vi "Tetra_TX-PROD_Setup.vi"() -> (0 "error out":errorcluster, 2 "Status":string="Skipping Setup of Power Supply\rDone !!!\rDONE!!\n\nSetting up PNA...\rRecalling PNA Setup:  Z:\\State Files\\TEST2.csa\rDONE!!!\rSkipping Spectrum Analyzer!!!\rSkipping Setting Up Temperature...\rSetup Complete !!!")   [LabVIEW 2018]
uses:
  <vilib>/Utility/error.llb/DialogType.ctl
  Tetra_Globals.vi
  Initialize References/Sequence Globals.vi
  Infrastructure/Test Parameter Globals_1.0.0.vi
  Initialize References/Station References Global.vi
  Infrastructure/Test Result File Name Global.vi
  <vilib>/Utility/file.llb/Read Delimited Spreadsheet (string).vi
  <vilib>/Utility/file.llb/Write Delimited Spreadsheet (string).vi
  Instruments/PNA/lib functions/Agilent ENA Series.lvlib
  Instruments/Agilent N5232A PNA-L/Labview Driver/Keysight PNA Series/Keysight PNA Series.lvlib
panel:
  out "IsPSA?(t)":bool
  out "Meas_S11?(t)":bool
  out "OUT_CAL_PATH(str)":string
  in  "ess_error":errorcluster
  in  "Tab Control":T1(tab)
  in  "Setup Chip (T)":bool=TRUE
  in  "Setup Power Supply (T)":bool=TRUE
  in  "Setup PNA (T)":bool=TRUE
  in  "Kill Teraterm":bool=TRUE
  in  "Setup Gantry(t)":bool=TRUE
  in  "Setup EXA(t)":bool=TRUE
  out "Success":bool
  out "MODE":bool
  out "COM PORT":string="COM4"
  out "RBW":string="3000"
  out "Avgs":u32=4
  out "SPAN":dbl=0.1
  out "REF_LVL":dbl=10.0
  out "PS1-1(V)":dbl=18.75
  out "PS1-1(A)":dbl=1.0
  out "PS1-2(V)":dbl=5.0
  out "PS1-2(A)":dbl=1.0
  out "Use PS1-2":bool=TRUE
  out "Use PS1-1":bool=TRUE
  out "EXA State File":string="Z:\\State Files\\State_0000.state"
  out "cmd;":string
  out "ATT_LVL":dbl=10.0
  out "TEMP":dbl=25.0
  out "TEMP?(t)":bool
  out "RF_FREQ":dbl=20.0
  out "f_ref":dbl=10.0
  out "REF_POWER":dbl=7.5
  out "Soak Time (s)":dbl=10.0 caption="Delay Time (s)"
  out "Ant":i16
  out "Gantry-Z":dbl
  out "GET_DET":bool
  out "OUT_CAL_PATH":path=path "C:/RageATE/Automated Tests/Tetra WAM/DVT/Cal Files/OUTPUT_CAL_080321-1118.csv"
  out "HORN_CAL_PATH":path
  out "RF_CAL_PATH":path
  out "git log":string="#RageATE gitlog: commit 9dda47de5732cf8fa6a9554b7d9ab91f125b5971\n#RageATE gitlog: Author: rick-rage <rick@ragesystems.com>\n#RageATE gitlog: Date:   Mon Aug 2 15:21:18 2021 -0400\n#RageATE gitlog: This Computer Name : CRANES\r\n\r\n"
  out "PNA State File":string="Z:\\State Files\\TEST2.csa"
  out "Text":refnum<vi>
  out "s11_path":path
  out "Pmic_FwRev":string
  out "i_mon":string
  out "rev":string="rdiv\r\n0)  sw3p6:   195 mA  3616 mV\r\n1)  sw5p5:    89 mA  5472 mV\r\n2) sw2p8a:   315 mA  2784 mV\r\n3) sw2p8b:   349 mA  2768 mV\r\n4)  sw2p4:  1458 mA  2288 mV\r\n5)  sw1p4:  1047 mA  1304 mV\r\n>"
  out "snic":string="#Family: 0x2D\n#Serial: 0x000036092740\r\n"
  in  "error in (no error)":errorcluster
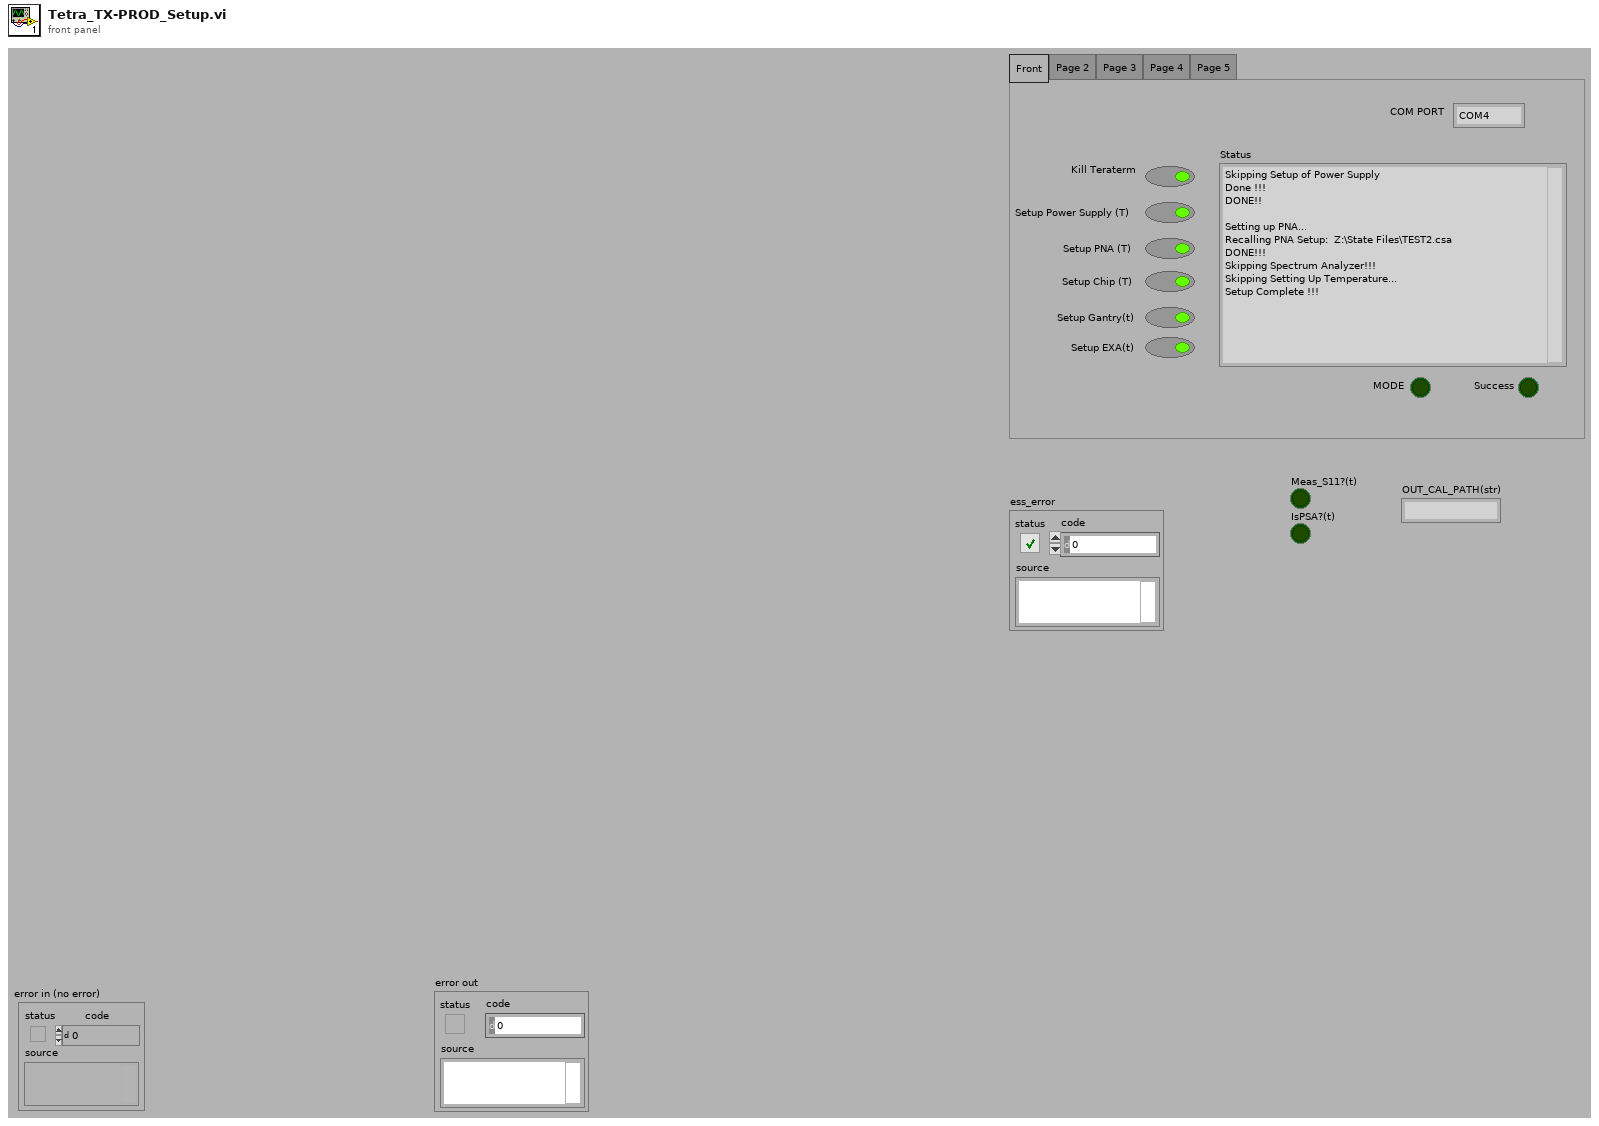
[diagram p1: front panel]
types:
  T1 = enum32{"Front", "Page 2", "Page 3", "Page 4", "Page 5"}
  T2 = typedef "DialogType.ctl" = u16
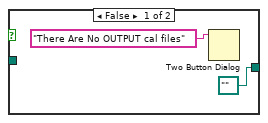
[diagram p2: hidden frame]
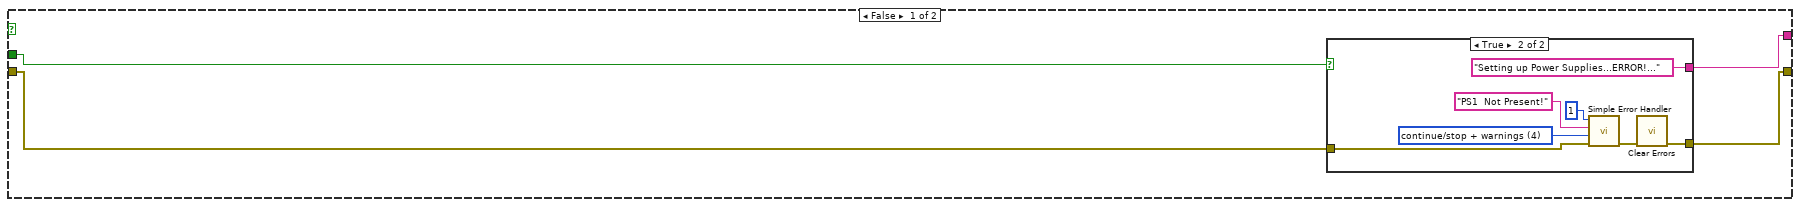
[diagram p6: hidden frame]
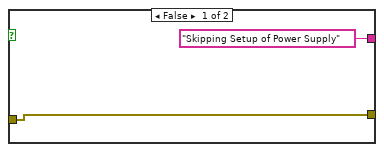
[diagram p7: hidden frame]
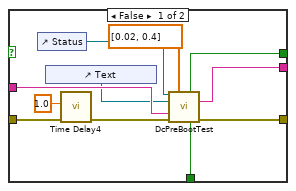
[diagram p8: hidden frame]
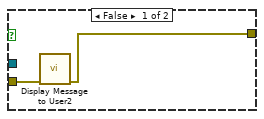
[diagram p10: hidden frame]
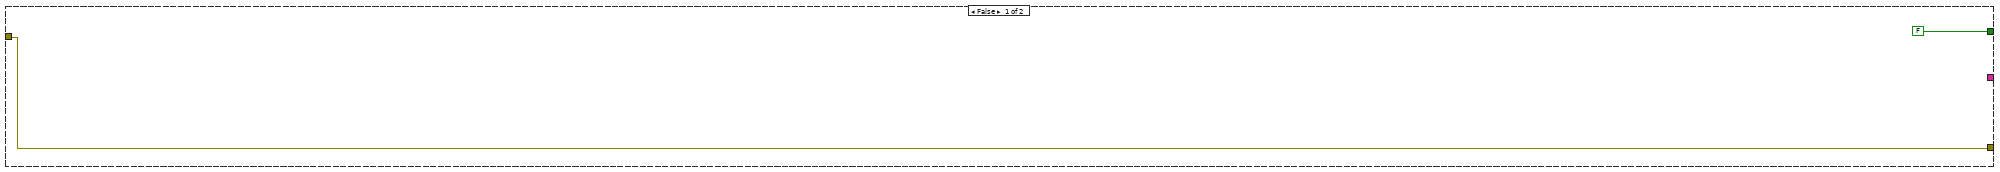
[diagram p11: hidden frame]
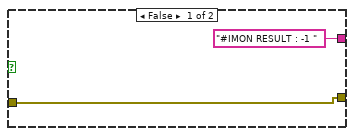
[diagram p12: hidden frame]
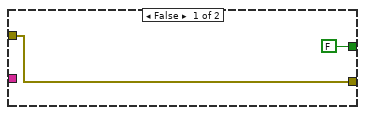
[diagram p13: hidden frame]
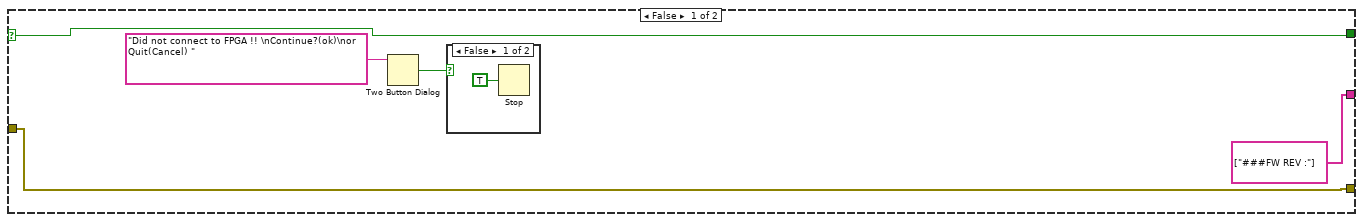
[diagram p14: hidden frame]
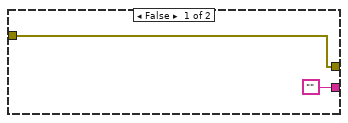
[diagram p16: hidden frame]
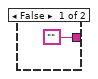
[diagram p18: hidden frame]
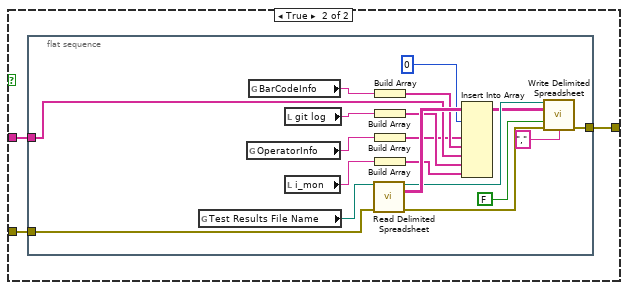
[diagram p19: hidden frame]
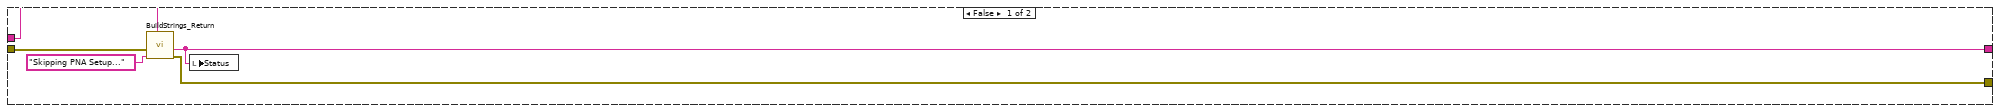
[diagram p20: hidden frame]
diagram:
  n1 = flat-sequence {
    tunnel: [w11] -> w1
    tunnel: [w51] -> w5
    tunnel: [w50] -> w4
    tunnel: w1 -> [w46]
    tunnel: w5 -> [w114]
    tunnel: w4 -> [w113]
    tunnel: [w265] -> w7
    tunnel: [w263] -> w6
    tunnel: w7 -> [w442]
    tunnel: w6 -> [w440]
    tunnel: [w436] -> w2
    tunnel: [w568] -> w3
    tunnel: w2 -> [w571]
    tunnel: w3 -> [w660]
    tunnel: [w655] -> w9
    tunnel: [w659] -> w8
    tunnel: w9 -> [w698]
    tunnel: w8 -> [w701]
    frame #0 {
      # "Kill TeraTerm"
      n2 = flat-sequence {
        tunnel: [w31] -> w11
        frame #0 {
          w29 = 1 items=["INPUT", "OUTPUT"] ("line index")
          (unwired) path "C:/RageATE/Automated Tests/Tetra WAM/PRODUCTION/Test Benches" ("base path")
          n3 = global read "Sequence Globals.vi" "DevSupportPath"() -> (w22:path)
          n4 = Strip Path(path=w22) -> (stripped path=w21:path)  [unwired: 1 out]
          n5 = Build Path(base path=w21, name or relative path=path "Automated Tests/Tetra WAM/PRODUCTION/Test Benches" ("base path")) -> (appended path=w19:path)
          n6 = global read "Sequence Globals.vi" "AppSupportPath"() -> (w25:path)
          n7 = global read "Tetra_Globals.vi" "TestBench_ID"() -> (w23:string)
          n8 = global read "Sequence Globals.vi" "IsRuntime?"() -> (w18:bool)
          n9 = Build Path(base path=w19, name or relative path=w23) -> (appended path=w33:path)
          n10 = Concatenate Strings(w23, " Calibration Files" ("name or relative path")) -> (w24:string)
          n11 = Build Path(base path=w33, name or relative path=w24) -> (appended path=w27:path)
          n12 = Select(t=w25, s=w18, f=w27) -> (s? t:f=w26:path)
          n13 = call "FindMostRecentCalFile.vi"("DIR_IN"=w26, "Test Bench (for filename match)"=w23, "line index"=w29, "IsRuntime?"=w18) -> ("Success?(t)"=w30:bool, "cal_path_out"=w28:path)  [unwired: 9 in, 1 out]
          n14 = case shown="True" w30 {
            tunnel: w28 -> [_ w36]
            tunnel: [path "" ("appended path") w36] -> w31
            frame False {
              n15 = Two Button Dialog(message="There Are No OUTPUT cal files") -> ()  [unwired: 2 in, 1 out]
            }
            frame True {
            }
          }
        }
      }
      n16 = global read "Sequence Globals.vi" "RageATE_Gitlog"() -> (→"git log":string)
      n17 = case shown="True" "Kill Teraterm" {
        tunnel: "error in (no error)" -> [w37 w39]
        tunnel: [w37 w38] -> w13
        tunnel: "taskkill /f /im ttermpro.exe" ("command line") -> [_ w41]
        frame False {
        }
        frame True {
          n18 = call <vilib>:"Clear Errors.vi"("error in (no error)"=w39) -> ("error out"=w40:errorcluster)  [unwired: 5 in, 1 out]
          n19 = call <vilib>:"System Exec.vi"("error in (no error)"=w40, "command line"=w41) -> ("error out"=w42:errorcluster)  [unwired: 6 in, 3 out]
          n20 = call "Time Delay2"("error in (no error)"=w42) -> ("error out"=w38:errorcluster)  [unwired: 10 in]
        }
      }
      n21 = property on="Status" class="Str"(error in=w13) -> (error out=w12:errorcluster, "Text"=→"Text":refnum<vi>)  [unwired: 1 in, 1 out]
      n22 = local write "error in (no error)"(w12) -> ()
    }
    frame #1 {
      n23 = local write "Success"(FALSE ("Success")) -> ()
      n24 = Path To String(path=w46) -> (string=w45:string)
      n25 = local write "Setup EXA(t)"("Setup EXA(t)") -> ()
      n26 = local write "Setup Gantry(t)"("Setup Gantry(t)") -> ()
      n27 = local write "Setup Chip (T)"("Setup Chip (T)") -> ()
      n28 = local write "Setup PNA (T)"("Setup PNA (T)") -> ()
      n29 = Concatenate Strings("#Out_Cal_Path: " ("string"), w45) -> (→"OUT_CAL_PATH(str)":string)
      n30 = local write "Setup Power Supply (T)"("Setup Power Supply (T)") -> ()
      n31 = global read "Test Parameter Globals_1.0.0.vi" "Input Constants Out"() -> (w51:string[])
      n32 = global read "Test Parameter Globals_1.0.0.vi" "Test Parameters"() -> (w50:string[][])
      "Status" <- ""
      "OUT_CAL_PATH" <- w46
    }
    frame #2 {
      w110 = 0 ("disabled index (col)")
      w99 = 11  # index
      n33 = Index Array(array=w113, index (row) #1=0 ("disabled index (row)"), index (col) #1=w110, index (row) #2=3 ("disabled index (row)"), index (col) #2=w110, index (row) #3=7 ("disabled index (row)"), index (col) #3=w110) -> (element #1=w108:string, element #2=w106:string, element #3=w104:string)
      n34 = Index Array(array=w114, index #6=w99, index #17=10 ("index")) -> (element #1=w122:string, element #2=w115:string, element #3=w82:string, element #4=w103:string, element #5=w77:string, element #6=w98:string, element #7=w84:string, element #8=w100:string, element #9=→"PNA State File":string, element #10=→"EXA State File":string, element #11=→"RBW":string, element #12=w91:string, element #13=w57:string, element #14=w89:string, element #15=w87:string, element #16=w86:string, element #17=w73:string)  [unwired: 15 in]
      "cmd;" <- w84
      n35 = call "TempControlWithBool.vi"("INPUT"=w108) -> ("out"=→"TEMP":dbl, "Valid(t)"=→"TEMP?(t)":bool)  [unwired: 6 in, 1 out]
      n36 = call "StringToNumberControlWithBool.vi"("String In"=w106) -> ("Number Out"=→"REF_POWER":dbl)  [unwired: 7 in, 1 out]
      n37 = call "StringToNumberControlWithBool.vi"("String In"=w104) -> ("Number Out"=w96:dbl)  [unwired: 7 in, 1 out]
      "RF_FREQ" <- w96
      n38 = global read "Sequence Globals.vi" "AppSupportPath"() -> (w67:path)
      n39 = global read "Sequence Globals.vi" "DevSupportPath"() -> (w65:path)
      n40 = global read "Sequence Globals.vi" "IsRuntime?"() -> (w69:bool)
      n41 = global write "Tetra_Globals.vi" "cmd;"(w84) -> ()
      n42 = Divide(x=w96, y=2.0) -> (x/y=→"f_ref":dbl)
      n43 = global read "Tetra_Globals.vi" "comport"() -> (w80:refnum<visa-resource-name>)
      n44 = Strip Path(path=w65) -> (stripped path=w64:path)  [unwired: 1 out]
      n45 = Empty String/Path?(string/path=w82) -> (empty?=w83:bool)
      n46 = call "StringToNumberControlWithBool.vi"("String In"=w103) -> ("NOT = 0"=→"MODE":bool)  [unwired: 7 in, 1 out]
      n47 = call "StringToNumberControlWithBool.vi"("String In"=w98) -> ("NOT = 0"=→"GET_DET":bool)  [unwired: 7 in, 1 out]
      n48 = call "StringToNumberControlWithBool.vi"("String In"=w100) -> ("Number Out"=→"Soak Time (s)":dbl)  [unwired: 7 in, 1 out]
      n49 = call "StringToNumberControlWithBool.vi"("String In"=w91) -> ("Number Out"=→"Avgs":dbl)  [unwired: 7 in, 1 out]
      n50 = call "StringToNumberControlWithBool.vi"("String In"=w89) -> ("Number Out"=→"SPAN":dbl)  [unwired: 7 in, 1 out]
      n51 = String To Path(string=w87) -> (path=→"RF_CAL_PATH":path)
      n52 = String To Path(string=w86) -> (path=w68:path)
      n53 = call "StringToNumberControlWithBool(x2).vi"("Seperator"=";", "string"=w73) -> ("NOT_0?"=→"Meas_S11?(t)":bool)  [unwired: 3 in, 6 out]
      n54 = Match Pattern(string=w122, regular expression=";") -> (before substring=w129:string, after substring=w128:string)  [unwired: 1 in, 2 out]
      n55 = Match Pattern(string=w115, regular expression=";") -> (before substring=w120:string, after substring=w119:string)  [unwired: 1 in, 2 out]
      n56 = call "StringToNumberControlWithBool(x2).vi"("Seperator"=";" ("regular expression"), "string"=w77) -> ("Num(2)"=w74:dbl, "Num"=→"Ant":dbl, "NOT_0?"=w76:bool)  [unwired: 3 in, 4 out]
      "Gantry-Z" <- w74
      n57 = Build Path(base path=w64, name or relative path="Automated Tests\\Tetra WAM\\PRODUCTION\\Test Benches\\Common") -> (appended path=w62:path)
      n58 = Strip Path(path=w68) -> (name=w61:string)  [unwired: 1 out]
      n59 = Select(t=w80, s=w83, f=w82) -> (s? t:f=→"COM PORT":refnum<visa-resource-name>)
      n60 = call "StringToNumberControlWithBool.vi"("String In"=w128) -> ("Number Out"=→"PS1-1(A)":dbl)  [unwired: 7 in, 1 out]
      n61 = call "StringToNumberControlWithBool.vi"("String In"=w119) -> ("Number Out"=→"PS1-2(A)":dbl)  [unwired: 7 in, 1 out]
      n62 = call "StringToNumberControlWithBool.vi"("String In"=w129) -> ("Number Out"=→"PS1-1(V)":dbl, "NOT = 0"=→"Use PS1-1":bool)  [unwired: 7 in]
      n63 = call "StringToNumberControlWithBool.vi"("String In"=w120) -> ("Number Out"=→"PS1-2(V)":dbl, "NOT = 0"=→"Use PS1-2":bool)  [unwired: 7 in]
      n64 = Build Path(base path=w62, name or relative path=w61) -> (appended path=w60:path)
      n65 = local write "Setup Gantry(t)"(w76) -> ()
      n66 = global write "Tetra_Globals.vi" "Gantry_Z"(w74) -> ()
      n67 = Build Path(base path=w67, name or relative path=w61) -> (appended path=w66:path)
      n68 = Select(t=w66, s=w69, f=w60) -> (s? t:f=→"HORN_CAL_PATH":path)
      n69 = call "StringToNumberControlWithBool(x2).vi"("Seperator"=";", "string"=w57) -> ("Num(2)"=→"ATT_LVL":dbl, "Num"=→"REF_LVL":dbl)  [unwired: 3 in, 5 out]
    }
    frame #3 {
      # "C:\\RageATE\\Automated Tests\\Tetra WAM\\PRODUCTION\\Test Benches\\Common\\Horn_Gain_121322.csv"
      n70 = flat-sequence {
        tunnel: w132 -> [w144]
        tunnel: [w143] -> w131
        frame #0 {
          n71 = local read "OUT_CAL_PATH"() -> (w147:path)
          n72 = call "GetCalData.vi"("Open new file T"=TRUE, "error in (no error)"=w144, "cal file path (dialog if empty)"=w147) -> ("error out"=w143:errorcluster, "array out"=w146:dbl[][])  [unwired: 3 in, 4 out]
          n73 = global write "Tetra_Globals.vi" "OUT_CAL"(w146) -> ()
        }
      }
      n74 = local read "error in (no error)"() -> (w132:errorcluster)
      n75 = case shown="True" TRUE {
        tunnel: w131 -> [w135 w137]
        tunnel: [w135 w136] -> w133
        frame False {
        }
        frame True {
          # "For Horn"
          n76 = flat-sequence {
            tunnel: w137 -> [w139]
            tunnel: [w138] -> w136
            frame #0 {
              n77 = local read "HORN_CAL_PATH"() -> (w142:path)
              n78 = call "GetCalData.vi"("Open new file T"=TRUE, "error in (no error)"=w139, "cal file path (dialog if empty)"=w142) -> ("error out"=w138:errorcluster, "array out"=w141:dbl[][])  [unwired: 3 in, 4 out]
              n79 = global write "Tetra_Globals.vi" "HORN_CAL"(w141) -> ()
            }
          }
        }
      }
      n80 = local write "error in (no error)"(w133) -> ()
    }
    frame #4 {
      n81 = global read "Station References Global.vi" "RF Switch Present?"() -> (w150:bool)
      n82 = local read "error in (no error)"() -> (w149:errorcluster)
      n83 = case shown="True" w150 {
        tunnel: w149 -> [w151 w155]
        tunnel: [w151 w154] -> w148
        frame False {
        }
        frame True {
          # "Set the Switch for TX"
          n84 = global read "Station References Global.vi" "RF Switch"() -> (w156:refnum<visa-resource-name>)
          n85 = call "RfSwitch_WAM_ATE.vi"("VISA_IN"=w156, "error in"=w155, "Source"=enum16{"RFSM", "PNA"}."PNA", "T/R"=enum16{"TX", "RX"}."TX") -> ("error out"=w154:errorcluster)  [unwired: 10 in, 1 out]
        }
      }
      n86 = local write "error in (no error)"(w148) -> ()
    }
    frame #5 {
    }
    frame #6 {
      n87 = local read "Setup Power Supply (T)"() -> (w163:bool)
      n88 = global read "Station References Global.vi" "PS1 Present?"() -> (w167:bool)
      n89 = local read "error in (no error)"() -> (w159:errorcluster)
      n90 = And(x=w167, y=w163) -> (x .and. y?=w165:bool)
      n91 = case shown="True" w165 {
        tunnel: [w171 w182] -> w158
        tunnel: w159 -> [w170 w184]
        tunnel: [w169 w181] -> w164
        tunnel: w163 -> [w168 _]
        frame False {
          n92 = case shown="True" w168 {
            tunnel: [w173 w176] -> w171
            tunnel: w170 -> [w173 w175]
            tunnel: ["Skipping Setup of Power Supply" "Setting up Power Supplies...ERROR!..."] -> w169
            frame False {
            }
            frame True {
              w178 = T2 4 items=["no dialog", "OK message", "continue or stop message", "OK message + warnings", "continue/stop + warnings"] ("type of dialog (OK msg:1)")
              n93 = call <vilib>:"Simple Error Handler.vi"("error code (no error:0)"=1, "error source (\" \")"="PS1  Not Present!" ("error source (\" \")"), "type of dialog (OK msg:1)"=w178, "error in (no error)"=w175) -> ("error out"=w177:errorcluster)  [unwired: 1 in, 4 out]
              n94 = call <vilib>:"Clear Errors.vi"("error in (no error)"=w177) -> ("error out"=w176:errorcluster)  [unwired: 5 in, 1 out]
            }
          }
        }
        frame True {
          n95 = for {
            N: 2 -> [w190]
            shift-right: [w193] -> w182
            shift-left: w184 -> [w202]
            i -> [w192]
            stop <- w195 continue-if-true
            n96 = stacked-sequence {
              tunnel: w202 -> [w257]
              tunnel: [w256] -> w199
              frame #0 {
                w241 = "PS1" ("SEL_PS")
                # "Conf I/V lim"
                n97 = local read "Text"() -> (w244:refnum<vi>)
                n98 = local read "PS1-1(V)"() -> (w251:dbl)
                n99 = local read "PS1-2(V)"() -> (w252:dbl)
                n100 = property class="Txt"(reference=w244, error in=w257, "Scroll Position"=i16 -1) -> (error out=w242:errorcluster)  [unwired: 1 out]
                n101 = local read "PS1-1(A)"() -> (w254:dbl)
                n102 = local read "PS1-2(A)"() -> (w253:dbl)
                n103 = global read "Station References Global.vi" "PS1"() -> (w255:refnum<visa-resource-name>)
                n104 = Build Array(w251, w252, 12.0 ("element")) -> (w246:dbl[])
                n105 = Build Array(w254, w253, 1.0 ("element")) -> (w247:dbl[])
                n106 = call "PS_SETUP_V-I-EN.vi"("VISA resource name"=w255, "SEL_PS"=w241, "error in (no error)"=w242, "Use Channel"=bool[] [FALSE, FALSE, FALSE, FALSE], "Current Lim"=w247, "Voltage Set"=w246) -> ("VISA resource name out"=w245:refnum<visa-resource-name>, "error out"=w249:errorcluster)  [unwired: 8 in]
                n107 = call "Time Delay"("error in (no error)"=w249) -> ("error out"=w240:errorcluster)  [unwired: 10 in]
                n108 = call "PS_SETUP_V-I-EN.vi"("VISA resource name"=w245, "SEL_PS"=w241, "error in (no error)"=w240, "Use Channel"=bool[] [TRUE, FALSE, FALSE, FALSE], "Current Lim"=w247, "Voltage Set"=w246) -> ("error out"=w256:errorcluster)  [unwired: 8 in, 1 out]
              }
            }
            n109 = Increment(x=w192) -> (x+1=w191:i32)
            n110 = Equal?(x=w190, y=w191) -> (x = y?=w189:bool)
            n111 = local read "Status"() -> (w187:string)
            n112 = local read "Text"() -> (w201:refnum<vi>)
            n113 = global read "Tetra_Globals.vi" "RevC(t)"() -> (w185:bool)
            n114 = call "BuildStrings_Return.vi"("Input String"=w187, "New String"="Power Supplies ON!", "error in (no error)"=w199, "reference"=w201) -> ("error out"=w198:errorcluster, "concatenated string"=w197:string)  [unwired: 5 in, 1 out]
            n115 = local write "Status"(w197) -> ()
            n116 = case shown="True" w185 {
              tunnel: w198 -> [w204 w223]
              tunnel: w197 -> [w213 w222]
              tunnel: [w212 w221] -> w196
              tunnel: [w211 w220] -> w195
              tunnel: [w210 w219] -> w194
              tunnel: [w207 w216] -> w186
              frame False {
                n117 = control-ref of="Status"() -> (w208:refnum<vi>)
                n118 = control-ref of="Text"() -> (w209:refnum<vi>)
                n119 = call "Time Delay4"("error in (no error)"=w204, "Delay Time (s)"=1.0) -> ("error out"=w205:errorcluster)  [unwired: 9 in]
                n120 = call "DcPreBootTest.vi"("String in"=w208, "lsl/hsl limit"=dbl[] [0.02, 0.4], "reference in"=w209, "concatenated string"=w213, "error in (no error)"=w205) -> ("DcLow?(t= low)"=w212:bool, "concatenated stringout"=w207:string, "FlagDC?(t)"=w211:bool, "error out"=w210:errorcluster)  [unwired: 7 in]
              }
              frame True {
                n121 = control-ref of="Status"() -> (w217:refnum<vi>)
                n122 = control-ref of="Text"() -> (w218:refnum<vi>)
                n123 = call "DcPreBootTest.vi"("String in"=w217, "lsl/hsl limit"=dbl[] [0.03, 0.25], "reference in"=w218, "concatenated string"=w222, "error in (no error)"=w223, "seconds to wait"=0.2) -> ("DcLow?(t= low)"=w221:bool, "concatenated stringout"=w216:string, "FlagDC?(t)"=w220:bool, "error out"=w219:errorcluster)  [unwired: 6 in]
              }
            }
            n124 = local write "Status"(w186) -> ()
            n125 = global read "Station References Global.vi" "PS1"() -> (w188:refnum<visa-resource-name>)
            n126 = case shown="True" w196 {
              selector: w196 -> [_ w228]
              tunnel: w194 -> [w224 w230]
              tunnel: [w224 w229] -> w193
              tunnel: w189 -> [_ w227]
              tunnel: w188 -> [_ w225]
              frame False {
              }
              frame True {
                n127 = And(x=w228, y=w227) -> (x .and. y?=w226:bool)
                n128 = case shown="True" w226 {
                  tunnel: w230 -> [w232 w236]
                  tunnel: [w231 w233] -> w229
                  tunnel: w225 -> [_ w237]
                  frame False {
                    n129 = call "Display Message to User2"("error in (no error)"=w232) -> ("error out"=w231:errorcluster)  [unwired: 9 in, 1 out]
                  }
                  frame True {
                    n130 = call "PS_SETUP_V-I-EN.vi"("VISA resource name"=w237, "error in (no error)"=w236, "Use Channel"=bool[] [FALSE, FALSE, FALSE, FALSE]) -> ("error out"=w234:errorcluster)  [unwired: 11 in, 1 out]
                    n131 = call "Display Message to User3"("error in (no error)"=w234) -> ("error out"=w233:errorcluster)  [unwired: 9 in, 1 out]
                    n132 = invoke class="VI" method="FP.Close"(error in=w233) -> ()  [unwired: 2 in, 3 out]
                  }
                }
              }
            }
          }
          n133 = local read "Status"() -> (w181:string)
        }
      }
      n134 = local read "Text"() -> (w160:refnum<vi>)
      n135 = call "BuildStrings_Return.vi"("seconds to wait"=1.0, "Input String"=w164, "New String"="Done !!!", "error in (no error)"=w158, "reference"=w160) -> ("error out"=w157:errorcluster, "concatenated string"=w162:string)  [unwired: 4 in, 1 out]
      n136 = local write "Status"(w162) -> ()
      n137 = local write "error in (no error)"(w157) -> ()
    }
    frame #7 {
      n138 = local read "error in (no error)"() -> (w259:errorcluster)
      n139 = local read "Setup Chip (T)"() -> (w258:bool)
      n140 = case shown="True" w258 {
        tunnel: [FALSE w295] -> w271
        tunnel: [w273 w294] -> w270
        tunnel: [_ w293] -> w267
        tunnel: w259 -> [w273 w292]
        frame False {
        }
        frame True {
          n141 = local read "Status"() -> (w283:string)
          n142 = local read "Text"() -> (w284:refnum<vi>)
          n143 = call "BuildStrings_Return.vi"("seconds to wait"=0.0, "Input String"=w283, "New String"="Booting up FPGA..." ("Delay text ..."), "error in (no error)"=w292, "reference"=w284) -> ("error out"=w282:errorcluster, "concatenated string"=w285:string)  [unwired: 4 in, 1 out]
          n144 = local write "Status"(w285) -> ()
          n145 = local read "Setup Chip (T)"() -> (w287:bool)
          n146 = call "Time Delay3"("error in (no error)"=w282, "Delay Time (s)"=10.0) -> ("error out"=w277:errorcluster)  [unwired: 9 in]
          n147 = local read "COM PORT"() -> (w286:string)
          n148 = case shown="True" w287 {
            tunnel: [FALSE ("Success") w320] -> w279
            tunnel: w277 -> [w307 w313]
            tunnel: [w307 w319] -> w280
            tunnel: w286 -> [_ w314]
            frame False {
            }
            frame True {
              n149 = VISA Close(VISA resource name=w314) -> (error out=w315:errorcluster)  [unwired: 1 in]
              n150 = local read "Status"() -> (w311:string)
              n151 = local read "Text"() -> (w312:refnum<vi>)
              n152 = call "Tetra Serial.vi"("COMPORT"=w314, "error in (no error)"=w315, "Command"="", "Open Ser(t)"=TRUE, "Close Ser(t)"=FALSE) -> ("Success"=w320:bool, "error out"=w319:errorcluster)  [unwired: 6 in, 3 out]
              n153 = call "BuildStrings_Return.vi"("Input String"=w311, "New String"="Opening Serial Port\n...Creating Global Ref", "error in (no error)"=w313, "reference"=w312) -> ("concatenated string"=w309:string)  [unwired: 5 in, 2 out]
              n154 = local write "Status"(w309) -> ()
            }
          }
          "Success" <- w279
          n155 = local read "Setup Chip (T)"() -> (w288:bool)
          n156 = global read "Tetra_Globals.vi" "RevC(t)"() -> (w274:bool)
          n157 = And(x=w274, y=w279) -> (x .and. y?=w275:bool)
          n158 = And(x=w288, y=w279) -> (x .and. y?=w289:bool)
          n159 = case shown="True" w275 {
            tunnel: [w297 w306] -> w281
            tunnel: w280 -> [w297 w305]
            tunnel: ["#IMON RESULT : -1 " ("string") w299] -> w278
            frame False {
            }
            frame True {
              n160 = control-ref of="Text"() -> (w304:refnum<vi>)
              n161 = local read "COM PORT"() -> (w298:string)
              n162 = control-ref of="Status"() -> (w303:refnum<vi>)
              n163 = call <vilib>:"Trim Whitespace.vi"("string"="#IMON_RESULT: ") -> ("trimmed string"=w301:string)  [unwired: 1 in]
              n164 = call "WAM-DC-HealthCheck.vi"("COMPORT"=w298, "error in (no error)"=w305, "reference in"=w303, "LVObjectRefNum in"=w304) -> ("error out"=w306:errorcluster, "i_mon"=w300:string)  [unwired: 5 in, 1 out]
              n165 = Concatenate Strings(w301, w300) -> (w299:string)
            }
          }
          "i_mon" <- w278
          n166 = case shown="True" w289 {
            selector: w289 -> [w324 w362]
            tunnel: w281 -> [w325 w339]
            tunnel: [w325 w360] -> w294
            tunnel: [w324 w362] -> w295
            tunnel: [string[] ["###FW REV :"] ("new element/subarray") w361] -> w293
            frame False {
              n167 = Two Button Dialog(message="Did not connect to FPGA !! \nContinue?(ok)\nor Quit(Cancel) ") -> (T button?=w322:bool)  [unwired: 2 in]
              n168 = case shown="False" w322 {
                frame False {
                  n169 = Stop(stop? (T)=TRUE) -> ()
                }
                frame True {
                }
              }
            }
            frame True {
              w331 = FALSE ("OpenSerial(t)")
              n170 = local read "MODE"() -> (w340:bool)
              n171 = case shown="True" w340 {
                tunnel: ["" ";wr reg 0x04 1032;" ("string")] -> w337
                tunnel: w339 -> [w363 w368]
                tunnel: [w363 w367] -> w338
                frame False {
                }
                frame True {
                  n172 = local read "Status"() -> (w370:string)
                  n173 = call "BuildStrings_Return.vi"("seconds to wait"=1.0, "Input String"=w370, "New String"="Setting Freq mode to Auto" ("Command"), "error in (no error)"=w368) -> ("error out"=w367:errorcluster, "concatenated string"=w366:string)  [unwired: 5 in, 1 out]
                  n174 = local write "Status"(w366) -> ()
                }
              }
              n175 = local read "GET_DET"() -> (w350:bool)
              n176 = case shown="True" w350 {
                tunnel: ["" "wr txm 0x49 0F" ("Command")] -> w341
                frame False {
                }
                frame True {
                }
              }
              n177 = local read "COM PORT"() -> (w327:string)
              n178 = Concatenate Strings("seq off;" ("Command"), w341, w337) -> (w343:string)
              n179 = call "SerRW-Array.vi"("COMPORT"=w327, "error in (no error)"=w338, "Command ( ; seperation)"=w343) -> ("comport"=w335:refnum<visa-resource-name>, "error out"=w336:errorcluster)  [unwired: 6 in, 5 out]
              n180 = call "Tetra_Rev.vi"("COMPORT"=w335, "error in (no error)"=w336) -> ("rev"=w357:string, "comport"=w355:refnum<visa-resource-name>, "error out"=w354:errorcluster)  [unwired: 9 in, 2 out]
              "rev" <- w357
              n181 = global read "Tetra_Globals.vi" "BarCodeESN"() -> (w328:string)
              n182 = call "Tetra_ReadESN.vi"("COMPORT"=w355, "BC_Esn"=w328, "error in (no error)"=w354) -> ("read"=w353:string, "esn"=w351:string, "error out"=w352:errorcluster)  [unwired: 8 in, 2 out]
              "snic" <- w353
              n183 = global write "Tetra_Globals.vi" "ESN"(w351) -> ()
              n184 = local read "cmd;"() -> (w346:string)
              n185 = call "ESNLookup.vi"("ESN"=w351, "error in"=w352) -> ("error out"=w334:errorcluster)  [unwired: 7 in, 2 out]
              n186 = Empty String/Path?(string/path=w346) -> (empty?=w348:bool)
              n187 = call "UCD_Device-Info.vi"("COMPORT"=w327, "error in (no error)"=w334, "OpenSerial(t)"=w331, "CloseSerial(t)"=w331) -> ("Pmic_FwRev"=w329:string, "comport"=w333:refnum<visa-resource-name>, "error out"=w332:errorcluster)  [unwired: 8 in, 1 out]
              "Pmic_FwRev" <- w329
              n188 = case shown="False" w348 {
                tunnel: w333 -> [w375 _]
                tunnel: w332 -> [w374 w376]
                tunnel: [w373 w376] -> w347
                tunnel: w346 -> [w372 _]
                frame False {
                  n189 = call "SerRW-Array.vi"("COMPORT"=w375, "error in (no error)"=w374, "Command ( ; seperation)"=w372) -> ("error out"=w373:errorcluster)  [unwired: 6 in, 6 out]
                }
                frame True {
                }
              }
              n190 = Concatenate Strings(w357, w353, "\r\n", w329) -> (w349:string)
              n191 = Concatenate Strings("FPGA Booted : " ("string"), w357, w349) -> (w358:string)
              n192 = local read "Status"() -> (w345:string)
              n193 = local read "Text"() -> (w344:refnum<vi>)
              n194 = call "BuildStrings_Return.vi"("Input String"=w345, "New String"=w358, "error in (no error)"=w347, "reference"=w344) -> ("error out"=w360:errorcluster, "concatenated string"=w359:string)  [unwired: 5 in, 1 out]
              n195 = local write "Status"(w359) -> ()
              n196 = Build Array(w349) -> (w361:string[])
            }
          }
        }
      }
      n197 = And(x=w271, y=FALSE) -> (x .and. y?=w269:bool)
      n198 = case shown="False" w269 {
        tunnel: w270 -> [w381 w416]
        tunnel: [w380 w415] -> w266
        tunnel: w267 -> [w379 w414]
        frame False {
          n199 = flat-sequence {
            tunnel: w381 -> [w399]
            tunnel: [w398] -> w380
            tunnel: w379 -> [_]
            frame #0 {
              w384 = "\r\n"
              n200 = local read "OUT_CAL_PATH(str)"() -> (w383:string)
              n201 = local read "git log"() -> (w395:string)
              n202 = global read "Test Parameter Globals_1.0.0.vi" "OperatorInfo"() -> (w396:string)
              n203 = global read "Test Parameter Globals_1.0.0.vi" "BarCodeInfo"() -> (w389:string)
              n204 = local read "Pmic_FwRev"() -> (w394:string)
              n205 = local read "i_mon"() -> (w390:string)
              n206 = local read "snic"() -> (w393:string)
              n207 = call <vilib>:"Trim Whitespace.vi"("string"=w395) -> ("trimmed string"=w386:string)  [unwired: 1 in]
              n208 = local read "rev"() -> (w387:string)
              n209 = global read "Test Result File Name Global.vi" "Test Results File Name"() -> (w382:path)
              n210 = flat-sequence {
                tunnel: w382 -> [w412]
                frame #0 {
                  w409 = "_S11"  # string
                  # "create s11 filename"
                  n211 = Path To String(path=w412) -> (string=w413:string)
                  n212 = Match Pattern(string=w413, regular expression=".csv") -> (before substring=w410:string, match substring=w406:string)  [unwired: 1 in, 2 out]
                  n213 = Concatenate Strings(w410, w409, w406) -> (w408:string)
                  n214 = String To Path(string=w408) -> (path=w407:path)
                  "s11_path" <- w407
                  n215 = global write "Tetra_Globals.vi" "s11_path"(w407) -> ()
                }
              }
              n216 = Concatenate Strings(w396, w384, w389, w387, w393, w394, w384, w390, w384, "#caladc -1" ("string"), w384, w386, w384, "#CaptureFileDirectory: <nocapture>" ("string"), w384, w383) -> (w392:string)
              n217 = call-poly <vilib>:"Read Delimited Spreadsheet.vi"("file path (dialog if empty)"=w382, "error in (no error)"=w399) -> ("new file path (Not A Path if cancelled)"=w404:path, "all rows"=w405:string[][], "error out"=w400:errorcluster)  [unwired: 8 in, 3 out]
              n218 = Build Array(w392) -> (w391:string[])
              n219 = Insert Into Array(array=w405, index (row)=0, new element=w391) -> (w402:string[][])  [unwired: 1 in]
              n220 = call-poly <vilib>:"Write Delimited Spreadsheet.vi"("file path (dialog if empty)"=w404, "2D data"=w402, "append to file? (new file:F)"=FALSE, "error in (no error)"=w400, "delimiter (\\t)"="," ("delimiter (\\t)")) -> ("error out"=w398:errorcluster)  [unwired: 9 in, 1 out]
            }
          }
        }
        frame True {
          n221 = flat-sequence {
            tunnel: w416 -> [w428]
            tunnel: [w427] -> w415
            tunnel: w414 -> [w425]
            frame #0 {
              n222 = global read "Test Result File Name Global.vi" "Test Results File Name"() -> (w435:path)
              n223 = global read "Test Parameter Globals_1.0.0.vi" "OperatorInfo"() -> (w420:string)
              n224 = global read "Test Parameter Globals_1.0.0.vi" "BarCodeInfo"() -> (w421:string)
              n225 = local read "git log"() -> (w424:string)
              n226 = local read "i_mon"() -> (w418:string)
              n227 = call-poly <vilib>:"Read Delimited Spreadsheet.vi"("file path (dialog if empty)"=w435, "error in (no error)"=w428) -> ("new file path (Not A Path if cancelled)"=w433:path, "all rows"=w434:string[][], "error out"=w429:errorcluster)  [unwired: 8 in, 3 out]
              n228 = Build Array(w421) -> (w422:string[])
              n229 = Build Array(w424) -> (w423:string[])
              n230 = Build Array(w420) -> (w419:string[])
              n231 = Build Array(w418) -> (w417:string[])
              n232 = Insert Into Array(array=w434, index (row)=0, new element #1=w419, new element #2=w422, new element #3=w425, new element #4=w423, new element #5=w417) -> (w431:string[][])  [unwired: 1 in]
              n233 = call-poly <vilib>:"Write Delimited Spreadsheet.vi"("file path (dialog if empty)"=w433, "2D data"=w431, "append to file? (new file:F)"=FALSE, "error in (no error)"=w429, "delimiter (\\t)"="," ("delimiter (\\t)")) -> ("error out"=w427:errorcluster)  [unwired: 9 in, 1 out]
            }
          }
        }
      }
      n234 = local read "Status"() -> (w261:string)
      n235 = local read "Text"() -> (w260:refnum<vi>)
      n236 = call "BuildStrings_Return.vi"("seconds to wait"=1.0, "Input String"=w261, "New String"="DONE!!\n\nSetting up PNA...", "error in (no error)"=w266, "reference"=w260) -> ("error out"=w265:errorcluster, "concatenated string"=w263:string)  [unwired: 4 in, 1 out]
      n237 = local write "Status"(w263) -> ()
    }
    frame #8 {
      n238 = global read "Station References Global.vi" "PNA Present?"() -> (w444:bool)
      n239 = local read "Setup PNA (T)"() -> (w445:bool)
      n240 = And(x=w445, y=w444) -> (x .and. y?=w443:bool)
      n241 = case shown="True" w443 {
        tunnel: w442 -> [w448 w497]
        tunnel: [w449 w486] -> w441
        tunnel: w440 -> [w451 w498]
        tunnel: [w447 w460] -> w439
        frame False {
          n242 = call "BuildStrings_Return.vi"("Input String"=w451, "New String"="Skipping PNA Setup...", "error in (no error)"=w448) -> ("error out"=w449:errorcluster, "concatenated string"=w447:string)  [unwired: 6 in, 1 out]
          n243 = local write "Status"(w447) -> ()
        }
        frame True {
          w470 = 0 items=["Normal", "SMC"] ("MODE")
          w469 = i64 1000000000 items=["GHz"=1000000000, "MHZ"=1000000] ("Units")
          w475 = 1 items=["Chopped", "Alternate"] ("Sweep Mode (0: Chopped)")
          w476 = 3 items=["Linear", "Logarithmic", "Power", "CW", "Segment", "Phase"] ("Sweep Type (0: Linear)")
          w489 = 1 ("Channel (1)")
          w499 = 1 items=["OFF", "ON"] ("STATE(0=OFF)")
          w501 = 3 items=["HOLD", "CONT", "GROUP", "SINGLE"]  # Mode
          w502 = 1  # Channel
          n244 = local read "PNA State File"() -> (w496:string)
          n245 = Concatenate Strings("Recalling PNA Setup:  " ("string"), w496) -> (w494:string)
          n246 = call "BuildStrings_Return.vi"("Input String"=w498, "New String"=w494, "error in (no error)"=w497) -> ("error out"=w491:errorcluster, "concatenated string"=w461:string)  [unwired: 6 in, 1 out]
          n247 = local write "Status"(w461) -> ()
          n248 = local read "Text"() -> (w493:refnum<vi>)
          n249 = property class="Txt"(reference=w493, error in=w491, "Scroll Position"=-1) -> (error out=w473:errorcluster)  [unwired: 1 out]
          n250 = for {
            N: 2 -> [_]
            tunnel: w496 -> [w537]
            tunnel: [w525] -> w464
            shift-right: [w526] -> w463
            shift-left: w473 -> [w536]
            n251 = global read "Station References Global.vi" "PNA"() -> (w535:refnum<visa-resource-name>)
            n252 = disable-structure shown="Enabled" {
              disable-tunnel: [w556 w558] -> w524
              disable-tunnel: w536 -> [w555 w558]
              disable-tunnel: [w554 w559] -> w532
              disable-tunnel: w535 -> [w553 w559]
              frame Disabled {
                n253 = call "N5232-PNA_ExecuteShortcut.vi"("Session In"=w553, "error in"=w555, "ShortcutNum"="3") -> ("Session Out"=w554:refnum<visa-resource-name>, "error out"=w556:errorcluster)  [unwired: 11 in]
              }
              frame Enabled {
              }
            }
            n254 = for {
              N: 1 -> [_]
              tunnel: w537 -> [w544]
              shift-right: [w542] -> w533
              shift-left: w532 -> [w541]
              shift-right: [w538] -> w534
              shift-left: w524 -> [w540]
              w543 = u16 0 items=["Entire Instrument State", "Segment Sweep Table", "Limit Table", "Power Sensor A", "Power Sensor B", "VBA Project", "Loss Compensation Table 1", "Loss Compensation Table 2", "Loss Compensation Table 3", "Loss Compensation Table 4", "Ripple Limit Table"] ("Data Type (0: Entire Instrument State)")
              n255 = call "Recall.vi"("error in (no error)"=w540, "File Name ()"=w544, "Data Type (0: Entire Instrument State)"=w543, "VISA resource name"=w541) -> ("error out"=w539:errorcluster, "VISA resource name out"=w542:refnum<visa-resource-name>)  [unwired: 6 in]
              n256 = call "Time Delay6"("error in (no error)"=w539) -> ("error out"=w538:errorcluster)  [unwired: 10 in]
            }
            n257 = case shown="No Error" w534 {
              selector: w534 -> [w561 w563]
              tunnel: w533 -> [w560 w566]
              tunnel: [w561 w562] -> w528
              tunnel: [w560 w565] -> w527
              frame No Error {
              }
              frame Error {
                n258 = call <vilib>:"Clear Errors.vi"("error in (no error)"=w563) -> ("error out"=w564:errorcluster)  [unwired: 5 in, 1 out]
                n259 = call "Reset.vi"("error in (no error)"=w564, "VISA resource name"=w566) -> ("error out"=w562:errorcluster, "VISA resource name out"=w565:refnum<visa-resource-name>)  [unwired: 8 in]
              }
            }
            n260 = call "ReadConfiguredPower.vi"("VISA resource name"=w527, "error in (no error)"=w528) -> ("RF Power ?(T: On)"=w531:bool, "VISA resource name out"=w529:refnum<visa-resource-name>, "error out"=w530:errorcluster)  [unwired: 11 in]
            n261 = case shown="False" w531 {
              tunnel: w529 -> [w549 w551]
              tunnel: w530 -> [w548 w552]
              tunnel: [w545 w552] -> w526
              tunnel: [w547 w551] -> w525
              frame False {
                n262 = call "Configure Power.vi"("VISA resource name"=w549, "Enable RF Power (T: Enable)"=TRUE, "error in (no error)"=w548) -> ("VISA resource name out"=w547:refnum<visa-resource-name>, "error out"=w546:errorcluster)  [unwired: 11 in]
                n263 = call "Time Delay5"("error in (no error)"=w546) -> ("error out"=w545:errorcluster)  [unwired: 10 in]
              }
              frame True {
              }
            }
          }
          n264 = local read "Meas_S11?(t)"() -> (w462:bool)
          n265 = case shown="True" w462 {
            tunnel: w464 -> [w511 _]
            tunnel: w463 -> [w510 w519]
            tunnel: [w510 w522] -> w456
            tunnel: [w511 w521] -> w457
            tunnel: w461 -> [w509 w518]
            tunnel: [w509 w516] -> w460
            frame False {
            }
            frame True {
              (unwired) FALSE ("Enable Auto Attenuation (T: Enable)")
              w520 = 3 items=["Hz", "KHz", "MHz", "GHz"] ("F(Units)")
              n266 = local read "s11_path"() -> (w512:path)
              n267 = call "BuildStrings_Return.vi"("seconds to wait"=2.0, "Input String"=w518, "New String"="\nMeasuring S11...", "error in (no error)"=w519) -> ("error out"=w514:errorcluster, "concatenated string"=w516:string)  [unwired: 5 in, 1 out]
              n268 = global read "Station References Global.vi" "PNA"() -> (w513:refnum<visa-resource-name>)
              n269 = call "GetSpData.vi"("VISA resource name"=w513, "S11 file path"=w512, "error in (no error)"=w514, "F(Units)"=w520) -> ("VISA resource name out"=w521:refnum<visa-resource-name>, "error out"=w522:errorcluster)  [unwired: 9 in, 1 out]
            }
          }
          n270 = call "Configure Sweep.vi"("Sweep Mode (0: Chopped)"=w475, "error in (no error)"=w456, "Sweep Type (0: Linear)"=w476, "VISA resource name"=w457) -> ("error out"=w477:errorcluster, "VISA resource name out"=w478:refnum<visa-resource-name>)  [unwired: 6 in]
          n271 = call "Configure Sweep Generation.vi"("Sweep Points (201)"=1, "error in (no error)"=w477, "VISA resource name"=w478) -> ("error out"=w455:errorcluster, "VISA resource name out"=w454:refnum<visa-resource-name>)  [unwired: 7 in]
          n272 = local read "f_ref"() -> (w471:dbl)
          n273 = call "PNA-L_SET-CWFREQ.vi"("Session In"=w454, "error in"=w455, "MODE"=w470, "FREQ"=w471, "Units"=w469, "CH"=1, "Source"=1) -> ("Session Out"=w453:refnum<visa-resource-name>, "error out"=w452:errorcluster)  [unwired: 10 in, 1 out]
          n274 = local read "REF_POWER"() -> (w481:dbl)
          n275 = call "PNA_MAIN_RF_STATE.vi"("Session In"=w453, "error in"=w452, "RO(T)"=FALSE, "STATE(0=OFF)"=w499) -> ("Session Out"=w484:refnum<visa-resource-name>, "error out"=w483:errorcluster)  [unwired: 9 in, 1 out]
          n276 = call "Configure Power.vi"("VISA resource name"=w484, "Enable Auto Attenuation (T: Enable)"=FALSE, "Attenuation (0 dB)"=0.0, "error in (no error)"=w483, "Power Level (0 dBm)"=w481) -> ("VISA resource name out"=w485:refnum<visa-resource-name>, "error out"=w482:errorcluster)  [unwired: 9 in]
          n277 = disable-structure shown="Disabled" {
            disable-tunnel: w502 -> [w508 _]
            disable-tunnel: w501 -> [w507 _]
            disable-tunnel: w485 -> [w506 _]
            disable-tunnel: w482 -> [w505 _]
            disable-tunnel: [w504 _] -> w466
            disable-tunnel: [w503 _] -> w465
            frame Disabled {
              n278 = call "PNA_SWEEP MODE.vi"("Mode"=w507, "Channel"=w508, "error in (no error)"=w505, "VISA resource name"=w506) -> ("error out"=w503:errorcluster, "VISA resource name out"=w504:refnum<visa-resource-name>)  [unwired: 6 in]
            }
            frame Enabled {
            }
          }
          n279 = call "Select Measurement.vi"("error in (no error)"=w465, "Measurement Name (CH1_S11_1)"="CH1_S11_1", "Channel (1)"=w489, "VISA resource name"=w466) -> ("error out"=w480:errorcluster, "VISA resource name out"=w479:refnum<visa-resource-name>)  [unwired: 6 in]
          n280 = call "Configure Marker_RageATE.vi"("Session In"=w479, "CH#"=w489, "MKR#"=1, "MKR ON(T)"=TRUE, "error in"=w480) -> ("error out"=w486:errorcluster)  [unwired: 9 in, 1 out]
        }
      }
      n281 = local read "Text"() -> (w437:refnum<vi>)
      n282 = call "BuildStrings_Return.vi"("Input String"=w439, "New String"="DONE!!!", "error in (no error)"=w441, "reference"=w437) -> ("error out"=w436:errorcluster, "concatenated string"=w438:string)  [unwired: 5 in, 1 out]
      n283 = local write "Status"(w438) -> ()
    }
    frame #9 {
      n284 = global read "Station References Global.vi" "Spectrum Analyzer Present?"() -> (w572:bool)
      n285 = local read "Setup EXA(t)"() -> (w569:bool)
      n286 = And(x=w572, y=w569) -> (x .and. y?=w570:bool)
      n287 = local read "Status"() -> (w567:string)
      n288 = case shown="True" w570 {
        tunnel: w571 -> [w576 w596]
        tunnel: [w577 w592] -> w568
        tunnel: w567 -> [w574 w590]
        frame False {
          n289 = local read "Text"() -> (w575:refnum<vi>)
          n290 = call "BuildStrings_Return.vi"("Input String"=w574, "New String"="Skipping Spectrum Analyzer!!!", "error in (no error)"=w576, "reference"=w575) -> ("error out"=w577:errorcluster, "concatenated string"=w573:string)  [unwired: 5 in, 1 out]
          n291 = local write "Status"(w573) -> ()
        }
        frame True {
          n292 = global read "Station References Global.vi" "Spectrum Analyzer Model"() -> (w581:string)
          n293 = Equal?(x=w581, y="E4447A") -> (x = y?=w579:bool)
          "IsPSA?(t)" <- w579
          n294 = global read "Station References Global.vi" "Spectrum Analyzer"() -> (w586:refnum<visa-resource-name>)
          n295 = local read "Text"() -> (w591:refnum<vi>)
          n296 = call "BuildStrings_Return.vi"("Input String"=w590, "New String"="Setting Up Spectrum Analyzer!!!", "error in (no error)"=w596, "reference"=w591) -> ("error out"=w589:errorcluster, "concatenated string"=w582:string)  [unwired: 5 in, 1 out]
          n297 = local read "EXA State File"() -> (w593:string)
          n298 = local write "Status"(w582) -> ()
          n299 = Empty String/Path?(string/path=w593) -> (empty?=w583:bool)
          n300 = call "Instrument Mode.vi"("SKIP(T)"=w579, "SET/GET"="SET", "error in"=w589, "Select INST"="INST SA", "Session In"=w586) -> ("error out"=w588:errorcluster, "Session Out"=w587:refnum<visa-resource-name>)  [unwired: 4 in, 1 out]
          n301 = case shown="False" w583 {
            tunnel: w587 -> [w651 w653]
            tunnel: w593 -> [w650 _]
            tunnel: w588 -> [w649 w652]
            tunnel: [w648 w652] -> w595
            tunnel: [w647 w653] -> w594
            frame False {
              n302 = call "EXA_RCL_STATE.vi"("FileName"=w650, "error in"=w649, "Session In"=w651) -> ("error out"=w648:errorcluster, "Session Out"=w647:refnum<visa-resource-name>)  [unwired: 7 in]
            }
            frame True {
            }
          }
          n303 = case shown="True" w583 {
            tunnel: w595 -> [w604 w624]
            tunnel: w594 -> [_ w626]
            tunnel: [w603 w635] -> w592
            frame False {
              n304 = local read "EXA State File"() -> (w598:string)
              n305 = Concatenate Strings("Load file  " ("New String"), w598, " to Spectrum Analyzer!!!" ("string")) -> (w602:string)
              n306 = local read "Status"() -> (w600:string)
              n307 = local read "Text"() -> (w606:refnum<vi>)
              n308 = call "BuildStrings_Return.vi"("Input String"=w600, "New String"=w602, "error in (no error)"=w604, "reference"=w606) -> ("error out"=w603:errorcluster, "concatenated string"=w599:string)  [unwired: 5 in, 1 out]
              n309 = local write "Status"(w599) -> ()
            }
            frame True {
              w622 = 1 items=["INTERNAL", "EXTERNAL", "SENSE(XA Series)", "PULS(XA Series)"] ("REF_SRC [INT|EXT]")
              w617 = 2 items=["Off", "Low Band", "Full Range"] ("Internal Preamp (0: Off)")
              w633 = u16 0 items=["OFF", "ON"] ("ON/OFF")
              w620 = FALSE ("Send OPC? (T)")
              w639 = u16 2 items=["Hz", "MHz", "GHz"] ("Freq Units")
              w640 = 1 items=["Clear Write", "Average", "Maximum Hold", "Minimum Hold"] ("Trace Type (0: Clear Write)")
              w641 = 0 items=["RBW AUTO OFF", "RBW AUTO ON"] ("RBW AUTO")
              n310 = local read "RF_FREQ"() -> (w638:dbl)
              n311 = call "SA_SET_REFSRC.vi"("Session In"=w626, "error in"=w624, "READ ONLY (T)"=FALSE, "REF_SRC [INT|EXT]"=w622) -> ("Session Out"=w625:refnum<visa-resource-name>, "error out"=w623:errorcluster)  [unwired: 9 in, 1 out]
              n312 = call "SA_SET_CF.vi"("Send OPC? (T)"=TRUE, "error in"=w623, "Freq Units"=w639, "SET CF ()"=w638, "Session In"=w625) -> ("error out"=w629:errorcluster, "Session Out"=w630:refnum<visa-resource-name>)  [unwired: 4 in, 1 out]
              n313 = local read "SPAN"() -> (w637:dbl)
              n314 = call "FREQ_SPAN.vi"("error in"=w629, "Span(MHz)"=w637, "Session In"=w630) -> ("error out"=w628:errorcluster, "Session Out"=w627:refnum<visa-resource-name>)  [unwired: 6 in, 1 out]
              n315 = local read "Avgs"() -> (w644:u32)
              n316 = call "SA_AVG.vi"("Session In"=w627, "AVG Count"=w644, "error in"=w628, "Trace Type (0: Clear Write)"=w640, "AVG Restart (T)"=w620, "Send OPC? (T)"=w620) -> ("Session Out"=w646:refnum<visa-resource-name>, "error out"=w645:errorcluster)  [unwired: 8 in]
              n317 = local read "RBW"() -> (w643:string)
              n318 = call "SA_RBW.vi"("Session In"=w646, "RBW(Hz)"=w643, "error in"=w645, "RO (T)"=FALSE, "RBW AUTO"=w641) -> ("Session Out"=w613:refnum<visa-resource-name>, "error out"=w614:errorcluster)  [unwired: 6 in, 3 out]
              n319 = local read "REF_LVL"() -> (w619:dbl)
              n320 = Greater Or Equal To 0?(x=w619) -> (x >= 0?=w618:bool)
              n321 = local read "ATT_LVL"() -> (w607:dbl)
              n322 = Select(t=0, s=w618, f=w617) -> (s? t:f=w615:i32)
              n323 = call "SA_PREAMP.vi"("VISA resource name"=w613, "error in (no error)"=w614, "Internal Preamp (0: Off)"=w615) -> ("VISA resource name out"=w612:refnum<visa-resource-name>, "error out"=w611:errorcluster)  [unwired: 11 in]
              n324 = call "REF_LEV.vi"("Session In"=w612, "RefLvl"=w619, "error in"=w611) -> ("Session Out"=w631:refnum<visa-resource-name>, "error out"=w610:errorcluster)  [unwired: 9 in, 2 out]
              n325 = call "SA_ATT.vi"("Session In"=w631, "ATT"=w607, "error in"=w610) -> ("Session Out"=w608:refnum<visa-resource-name>, "error out"=w609:errorcluster)  [unwired: 9 in, 2 out]
              n326 = call "SWEEP_CONT.vi"("Session In"=w608, "OPC?"=TRUE, "ON/OFF"=w633, "error in"=w609, "RO (T)"=FALSE) -> ("error out"=w635:errorcluster)  [unwired: 8 in, 2 out]
            }
          }
        }
      }
    }
    frame #10 {
      n327 = global read "Station References Global.vi" "Oven Present?"() -> (w658:bool)
      n328 = local read "TEMP?(t)"() -> (w656:bool)
      n329 = And(x=w656, y=w658) -> (x .and. y?=w657:bool)
      n330 = local read "Status"() -> (w654:string)
      n331 = case shown="False" w657 {
        tunnel: w660 -> [w667 w688]
        tunnel: w654 -> [w665 w687]
        tunnel: [w661 w681] -> w659
        tunnel: w656 -> [w666 _]
        tunnel: [w663 w678] -> w655
        frame False {
          n332 = disable-structure shown="Disabled" {
            frame Disabled {
              n333 = global write "Station References Global.vi" "Oven Present?"(FALSE ("Oven Present?")) -> ()
            }
            frame Enabled {
            }
          }
          n334 = call "Display Message to User"("error in (no error)"=w667, "Enable"=w666) -> ("error out"=w662:errorcluster, "Cancel"=w664:bool)  [unwired: 8 in]
          n335 = Stop(stop? (T)=w664) -> ()
          n336 = case shown="False" w664 {
            tunnel: w665 -> [w673 w676]
            tunnel: [w672 w676] -> w661
            tunnel: [w671 w675] -> w663
            tunnel: w662 -> [w670 w675]
            frame False {
              n337 = local read "Text"() -> (w669:refnum<vi>)
              n338 = call "BuildStrings_Return.vi"("Input String"=w673, "New String"="Skipping Setting Up Temperature...", "error in (no error)"=w670, "reference"=w669) -> ("error out"=w671:errorcluster, "concatenated string"=w672:string)  [unwired: 5 in, 1 out]
            }
            frame True {
            }
          }
          n339 = local write "Status"(w661) -> ()
        }
        frame True {
          n340 = local read "Text"() -> (w677:refnum<vi>)
          n341 = call "BuildStrings_Return.vi"("Input String"=w687, "New String"="Setting Up Temperature...", "error in (no error)"=w688, "reference"=w677) -> ("error out"=w685:errorcluster, "concatenated string"=w681:string)  [unwired: 5 in, 1 out]
          n342 = local write "Status"(w681) -> ()
          n343 = global read "Station References Global.vi" "Oven"() -> (w686:refnum<visa-resource-name>)
          n344 = local read "TEMP"() -> (w684:dbl)
          n345 = call "PM9 Set Temp and Wait.vi"("VISA"=w686, "Error In"=w685, "Accuracy +/-"=2.0, "Set Point"=w684, "RO(t)"=FALSE, "Min (-1 for cont.)"=0.1 ("Min"), "close session(t)"=TRUE) -> ("error out"=w678:errorcluster)  [unwired: 9 in, 3 out]
        }
      }
    }
    frame #11 {
      n346 = global read "Station References Global.vi" "Gantry Present?"() -> (w693:bool)
      n347 = local read "Setup Gantry(t)"() -> (w695:bool)
      n348 = local read "Text"() -> (w697:refnum<vi>)
      n349 = And(x=w695, y=w693) -> (x .and. y?=w694:bool)
      n350 = case shown="True" w694 {
        tunnel: "ess_error" -> [w703 w707]
        tunnel: [w703 w714] -> w691
        frame False {
        }
        frame True {
          w709 = 21.0  # z ref
          w710 = u16 0 items=["Inches", "cm"] ("Zunits")
          n351 = global read "Station References Global.vi" "Gantry"() -> (w708:refnum<visa-resource-name>)
          n352 = for {
            N: 2 -> [_]
            tunnel: w708 -> [w724]
            shift-right: [w719] -> w706
            shift-left: w707 -> [w723]
            tunnel: [w716] -> w704
            stop <- w717 stop-if-true
            w722 = TRUE ("Open Serial")
            n353 = call "WAM_ESS.vi"("VISA resource name"=w724, "error in (no error)"=w723, "Open Serial"=w722, "Test Running (T)"=w722, "Close Serial"=w722) -> ("Enabled(T-RO)"=w721:bool, "FH_NOT(T)"=w720:bool, "VISA resource name out"=w715:refnum<visa-resource-name>, "error out"=w718:errorcluster)  [unwired: 7 in]
            n354 = And(x=w721, y=w720) -> (x .and. y?=w717:bool)
            n355 = case shown="False" w717 {
              tunnel: [w733 w735] -> w719
              tunnel: w718 -> [w731 w735]
              tunnel: [w728 w734] -> w716
              tunnel: w715 -> [w727 w734]
              frame False {
                w725 = TRUE ("Close Serial")
                w726 = u16 1 items=["Disable Driver", "Enable Driver", "Read Driver Status"] ("Driver-Func")
                n356 = call "Prompt User for Input"("error in (no error)"=w731) -> ("RESET"=w730:bool, "error out"=w732:errorcluster)  [unwired: 17 in]
                n357 = Not(x=w730) -> (.not. x?=w729:bool)
                n358 = Stop(stop? (T)=w729) -> ()
                n359 = call "Gantry_Driver.vi"("VISA resource name"=w727, "error in (no error)"=w732, "Open Serial"=w725, "Driver-Func"=w726, "Close Serial"=w725) -> ("VISA resource name out"=w728:refnum<visa-resource-name>, "error out"=w733:errorcluster)  [unwired: 11 in, 2 out]
              }
              frame True {
              }
            }
          }
          n360 = local read "Gantry-Z"() -> (w711:dbl)
          n361 = local read "Ant"() -> (w712:i16)
          n362 = call "Gantry.vi"("COMPORT"=w704, "error in (no error)"=w706, "Antenna Select"=w712, "z ref"=w709, "Write(reads antenna co-ords when off)"=TRUE, "z"=w711, "Zunits"=w710) -> ("error out"=w714:errorcluster)  [unwired: 12 in]
        }
      }
      n363 = call "BuildStrings_Return.vi"("seconds to wait"=1.0, "Input String"=w701, "New String"="Setup Complete !!!", "error in (no error)"=w698, "reference"=w697) -> ("error out"=w696:errorcluster, "concatenated string"=w702:string)  [unwired: 4 in, 1 out]
      "error out" <- w696
      n364 = local write "Status"(w702) -> ()
      n365 = local write "ess_error"(w691) -> ()
      n366 = Merge Errors(w696, w691) -> (w692:errorcluster)
      n367 = global write "Test Parameter Globals_1.0.0.vi" "Setup.vi Error"(w692) -> ()
    }
  }
